vi "Pockels modulation-Gen AO seq for funct img.vi"(7 "Run as sub-VI":bool, 11 "Setup/Logging queue element":T8={"Imaging Protocol"=enum."Live Imaging", "Number of Trials"=0, "Frame Size"=512, "# Averaged frames"=0, "Dwell time (us)"=0.0, "Index of Z-plane"=0, "Timelapse?"=FALSE, "Logging process is active"=FALSE, "Speed logging enabled"=FALSE, "tdms file ref"=refnum, "path"=path "", "Trial Number"=0, "Expected # points acquired"=FALSE, "Manually stopped"=FALSE, "Last trial"=FALSE, "Ch0 data"=[], "Ch1 data"=[], "Ref Data"=[], "Ref Frame Time"=[], "Image Time"=[], "Continuous Time"=[], "Ref X Length"=0, "Ref Y Length"=0, "# Ref Averaged frames"=0, "Ref Dwell time (us)"=0.0, "Points acquired"={"Ch0 last trial"=0, "Ch1 last trial"=0, "All trials"=0}, "HW Timings File"=refnum} {"Ref Dwell time (us)" format="%#.6g"; "Frame Size" items=["100X100"=100, "128X128"=128, "200X200"=200, "256X256"=256, "512X512"=512, "1024x1024"=1024, "2048x2048"=2048]; "Dwell time (us)" format="%#.6g"}) -> (1 "Pockels modulation sequence":dbl[](array[numeric])=[0.0, 0.0, 0.0, 0.0, 0.0, 0.0, 0.0, 0.0, 0.0, 0.0, 0.0, 0.0, 0.0, 0.0, 0.0, 0.0, 0.0, 0.0, 0.0, 0.0, 0.0, 0.0, 0.48, 0.48, 0.48, 0.48, 0.48, 0.48, 0.0, 0.0, 0.0, 0.0, 0.0, 0.0, 0.0, 0.0, 0.0, 0.0, 0.0, 0.0, 0.0, 0.0, 0.0, 0.0, 0.0, 0.0, 0.5308080000000001, 0.5308080000000001, 0.5308080000000001, 0.5308080000000001, 0.5308080000000001, 0.5308080000000001, 0.0, 0.0, 0.0, 0.0, 0.0, 0.0, 0.0, 0.0, 0.0, 0.0, 0.0, 0.0, 0.0, 0.0, 0.0, 0.0, 0.0, 0.0, 0.0, 0.586992, 0.586992, 0.586992, 0.586992, 0.586992, 0.586992, 0.0, 0.0, 0.0, 0.0, 0.0, 0.0, 0.0, 0.0, 0.0, 0.0, 0.0, 0.0, 0.0, 0.0, 0.0, 0.0, 0.0, 0.0, 0.649124, 0.649124, 0.649124, 0.649124, 0.649124, 0.649124, 0.0, 0.0, 0.0, 0.0, 0.0, 0.0, 0.0, 0.0, 0.0, 0.0, 0.0, 0.0, 0.0, 0.0, 0.0, 0.0, 0.0, 0.0, 0.0, 0.717834, 0.717834, 0.717834, 0.717834, 0.717834, 0.717834, 0.0, 0.0, 0.0, 0.0, 0.0, 0.0, 0.0, 0.0, 0.0, 0.0, 0.0, 0.0, 0.0, 0.0, 0.0, 0.0, 0.0, 0.0, 0.793814, 0.793814, 0.793814, 0.793814, 0.793814, 0.793814, 0.0, 0.0, 0.0, 0.0, 0.0, 0.0, 0.0, 0.0, 0.0, 0.0, 0.0, 0.0, 0.0, 0.0, 0.0, 0.0, 0.0, 0.0, 0.0, 0.0, 0.0, 0.0, 0.0, 0.0, 0.0, 0.0, 0.0, 0.0, 0.0, 0.0, 0.0, 0.0, 0.0, 0.0, 0.0, 0.0, 0.0, 0.0, 0.0, 0.0, 0.0, 0.0, 0.0, 0.970756, 0.970756, 0.970756, 0.970756, 0.970756], 2 "Sampling period (us)":dbl=1e-06, 3 "Sequence length (ms)":dbl=198.0 format="%#_g ms", 4 "Sequence length (points)":i32=198 format="%.0f points")   [LabVIEW 2020]
uses:
  Typedefs/Logging queue element.ctl
  Typedefs/Imaging Protocols enum.ctl
  Typedefs/Frame Size.ctl
  Typedefs/Acquired points count.ctl
  Typedefs/Pockels-Funct acq simulation inputs cluster.ctl
  Typedefs/Controls/AOL_Globals.ctl
  Typedefs/AOL modes.ctl
  Typedefs/Plane Mode.ctl
  Typedefs/Functional Mode.ctl
  <vilib>/GPower/Comparison/Library/IsOdd/IsOddI32.vi
  <vilib>/GPower/Comparison/GPComparison.lvlib
panel:
  out "Last AOL_Globals used":T1={"Imaging Protocol"=enum."AOL Z-Stack", "Number of POI"=0, "Number of Miniscans"=0, "Number of Trials"=0, "Number of Cycles "=0, "# Averaged Frames"=0, "Laser power (%)"=0, "Pockels (V)"=0.0, "Acquisition Length (sec)"=0.0, "Fill time (us)"=0.0, "POI Dwell time (us)"=0.0, "Miniscan Dwell time per pixel (us)"=0.0, "PMT 1"=0.0, "PMT 2"=0.0, "Back Apperture (mA)"=200.0, "Frame Size"=0, "Center Frequency"=0.0, "Field of View (um)"=175.0, "Field of View (norm)"=0.0, "DwellTime (us)"=0.0, "Ref Dwell Time (us)"=0.0, "Wavelength (nm)"=0.0, "Zoom"=0.0, "AOL Z"=0.0, "AOL Mode"=enum."Raster", "GridXY"=0.0, "GridZ"=0.0, "TriggerPeriod (sec)"=0.0, "Number of Pixels in Miniscan"=0, "Experiment folder path"=path "", "X centre"=0.0, "Y centre"=0.0, "Angle (degrees)"=0.0, "Angle Xs (degrees)"=0.0, "Angle Ys (degrees)"=0.0, "Plane Mode"=0, "Threshold"=[], "Regenerate Chirps"=FALSE, "Rectangle ROI length (pixels)"=0, "Rectangle ROI height (pixels)"=0, "AOD fill"=4900, "StartupDelay"=0, "Samples Wait after Trigger"=5080, "Slip Cycle"=600000, "Add Cycle"=TRUE, "Functional Mode"=enum."Point", "Z Start"=0.0, "Z Stop"=0.0, "# Planes"=0, "Total Pixels"=0, "Variable Miniscan Pixels"=[], "Use Variable Length"=FALSE, "Use Variable Resolution"=FALSE, "Laser power (%) at Z Start"=0, "Laser power (%) at Z Stop"=0, "Ref Z Step"=0} {"Angle Ys (degrees)" format="%#.6g"; "Angle Xs (degrees)" format="%#.6g"; "Plane Mode" items=["XY Plane", "XZ Plane", "YZ Plane", "arbitraryplane"]; "Frame Size" items=["100X100"=100, "128X128"=128, "200X200"=200, "256X256"=256, "512X512"=512, "1024x1024"=1024, "2048x2048"=2048]; "Back Apperture (mA)" format="%#.6g"; "Pockels (V)" format="%#.6g"; "PMT 2" format="%#.6g"; "PMT 1" format="%#.6g"; "Angle (degrees)" format="%#.6g"; "POI Dwell time (us)" format="%#.6g"}
  in  "Temp Patch":bool=TRUE
  out "Loop":i32
  in  "Simulation inputs cluster":T7={"Dwell time (us) -Manual"=4.2, "Simulated number of POI"=80, "Bypass"=TRUE, "Movement Correction"=TRUE, "Ref_dwellTime"=0.1, "Ref X-pixels-per-line(Npxr)"=13, "Ref Y-lines-per-image(Npyr)"=12, "Ref Z-Plane index"=30, "Pockels \"Low\" time (us)"=20.0, "AO Sample Clock Rate (samples/sec)"=1000000.0, "Target time between mov.cor. ref triggers (ms)"=2.0, "Control system simulated waveform"=TRUE} {"AO Sample Clock Rate (samples/sec)" format="%#_6f"; "Dwell time (us) -Manual" min=0.05 max=10.0 step=0.1 format="%#.1fus"}
  out "Ref Scan Cycles":i32
  out "Adjusted time between ref \ntriggers sent to the FPGA (ms)":dbl
  in  "Pockels turn ON at least this number of us before fill time completion":dbl=4.0 min=0.05 max=10.0 step=1.0 format="%#.1fus"
  out "Number of POI":i32=8
  out "Cursor distance (us)":dbl=2.0 format="%#_g us"
  out "AO card sampling interval (us)":dbl=1.0 format="%#_13g us"
  out "Fill time (us)":dbl=24.4 format="%#_g us"
  in  "Pockels stay ON for at least this number of us after dwell time":dbl=2.0 min=0.5 max=10.0 step=1.0 format="%#.1fus"
  out "Graph":waveform(dbl)[](graph)=[{"t0"=timestamp(0 s since 1904-01-01), "dt"=0.05, "Y"=array[4561 elements]}, {"t0"=timestamp(0 s since 1904-01-01), "dt"=1.0, "Y"=[0.0, 0.0, 0.0, 0.0, 0.0, 0.0, 0.0, 0.0, 0.0, 0.0, 0.0, 0.0, 0.0, 0.0, 0.0, 0.0, 0.0, 0.0, 0.0, 0.0, 2.0, 2.0, 2.0, 2.0, 2.0, 2.0, 2.0, 2.0, 2.0, 2.0, 2.0, 2.0, 0.0, 0.0, 0.0, 0.0, 0.0, 0.0, 0.0, 0.0, 0.0, 0.0, 0.0, 0.0, 0.0, 0.0, 0.0, 0.0, 0.0, 2.0, 2.0, 2.0, 2.0, 2.0, 2.0, 2.0, 2.0, 2.0, 2.0, 2.0, 0.0, 0.0, 0.0, 0.0, 0.0, 0.0, 0.0, 0.0, 0.0, 0.0, 0.0, 0.0, 0.0, 0.0, 0.0, 0.0, 0.0, 2.0, 2.0, 2.0, 2.0, 2.0, 2.0, 2.0, 2.0, 2.0, 2.0, 2.0, 2.0, 0.0, 0.0, 0.0, 0.0, 0.0, 0.0, 0.0, 0.0, 0.0, 0.0, 0.0, 0.0, 0.0, 0.0, 0.0, 0.0, 0.0, 2.0, 2.0, 2.0, 2.0, 2.0, 2.0, 2.0, 2.0, 2.0, 2.0, 2.0, 0.0, 0.0, 0.0, 0.0, 0.0, 0.0, 0.0, 0.0, 0.0, 0.0, 0.0, 0.0, 0.0, 0.0, 0.0, 0.0, 0.0, 2.0, 2.0, 2.0, 2.0, 2.0, 2.0, 2.0, 2.0, 2.0, 2.0, 2.0, 2.0, 0.0, 0.0, 0.0, 0.0, 0.0, 0.0, 0.0, 0.0, 0.0, 0.0, 0.0, 0.0, 0.0, 0.0, 0.0, 0.0, 0.0, 2.0, 2.0, 2.0, 2.0, 2.0, 2.0, 2.0, 2.0, 2.0, 2.0, 2.0, 0.0, 0.0, 0.0, 0.0, 0.0, 0.0, 0.0, 0.0, 0.0, 0.0, 0.0, 0.0, 0.0, 0.0, 0.0, 0.0, 0.0, 2.0, 2.0, 2.0, 2.0, 2.0, 2.0, 2.0, 2.0, 2.0, 2.0, 2.0, 2.0, 0.0, 0.0, 0.0, 0.0, 0.0, 0.0, 0.0, 0.0, 0.0, 0.0, 0.0, 0.0, 0.0, 0.0, 0.0, 0.0, 0.0, 2.0, 2.0, 2.0, 2.0, 2.0, 2.0, 2.0]}]
  # "NOTE!\nThe always-simulated \"Control System\" signal may be wrong when Movement Correction is active as it won't include the reference frame time if\nthe number of POI result in very short original cycle time."
  # "<--- The pockels is an analogue signal which takes 3us to reach its value. Using 4us here ensures that the moment when data is acquired the pockels modulation signal has already reached its nominal value."
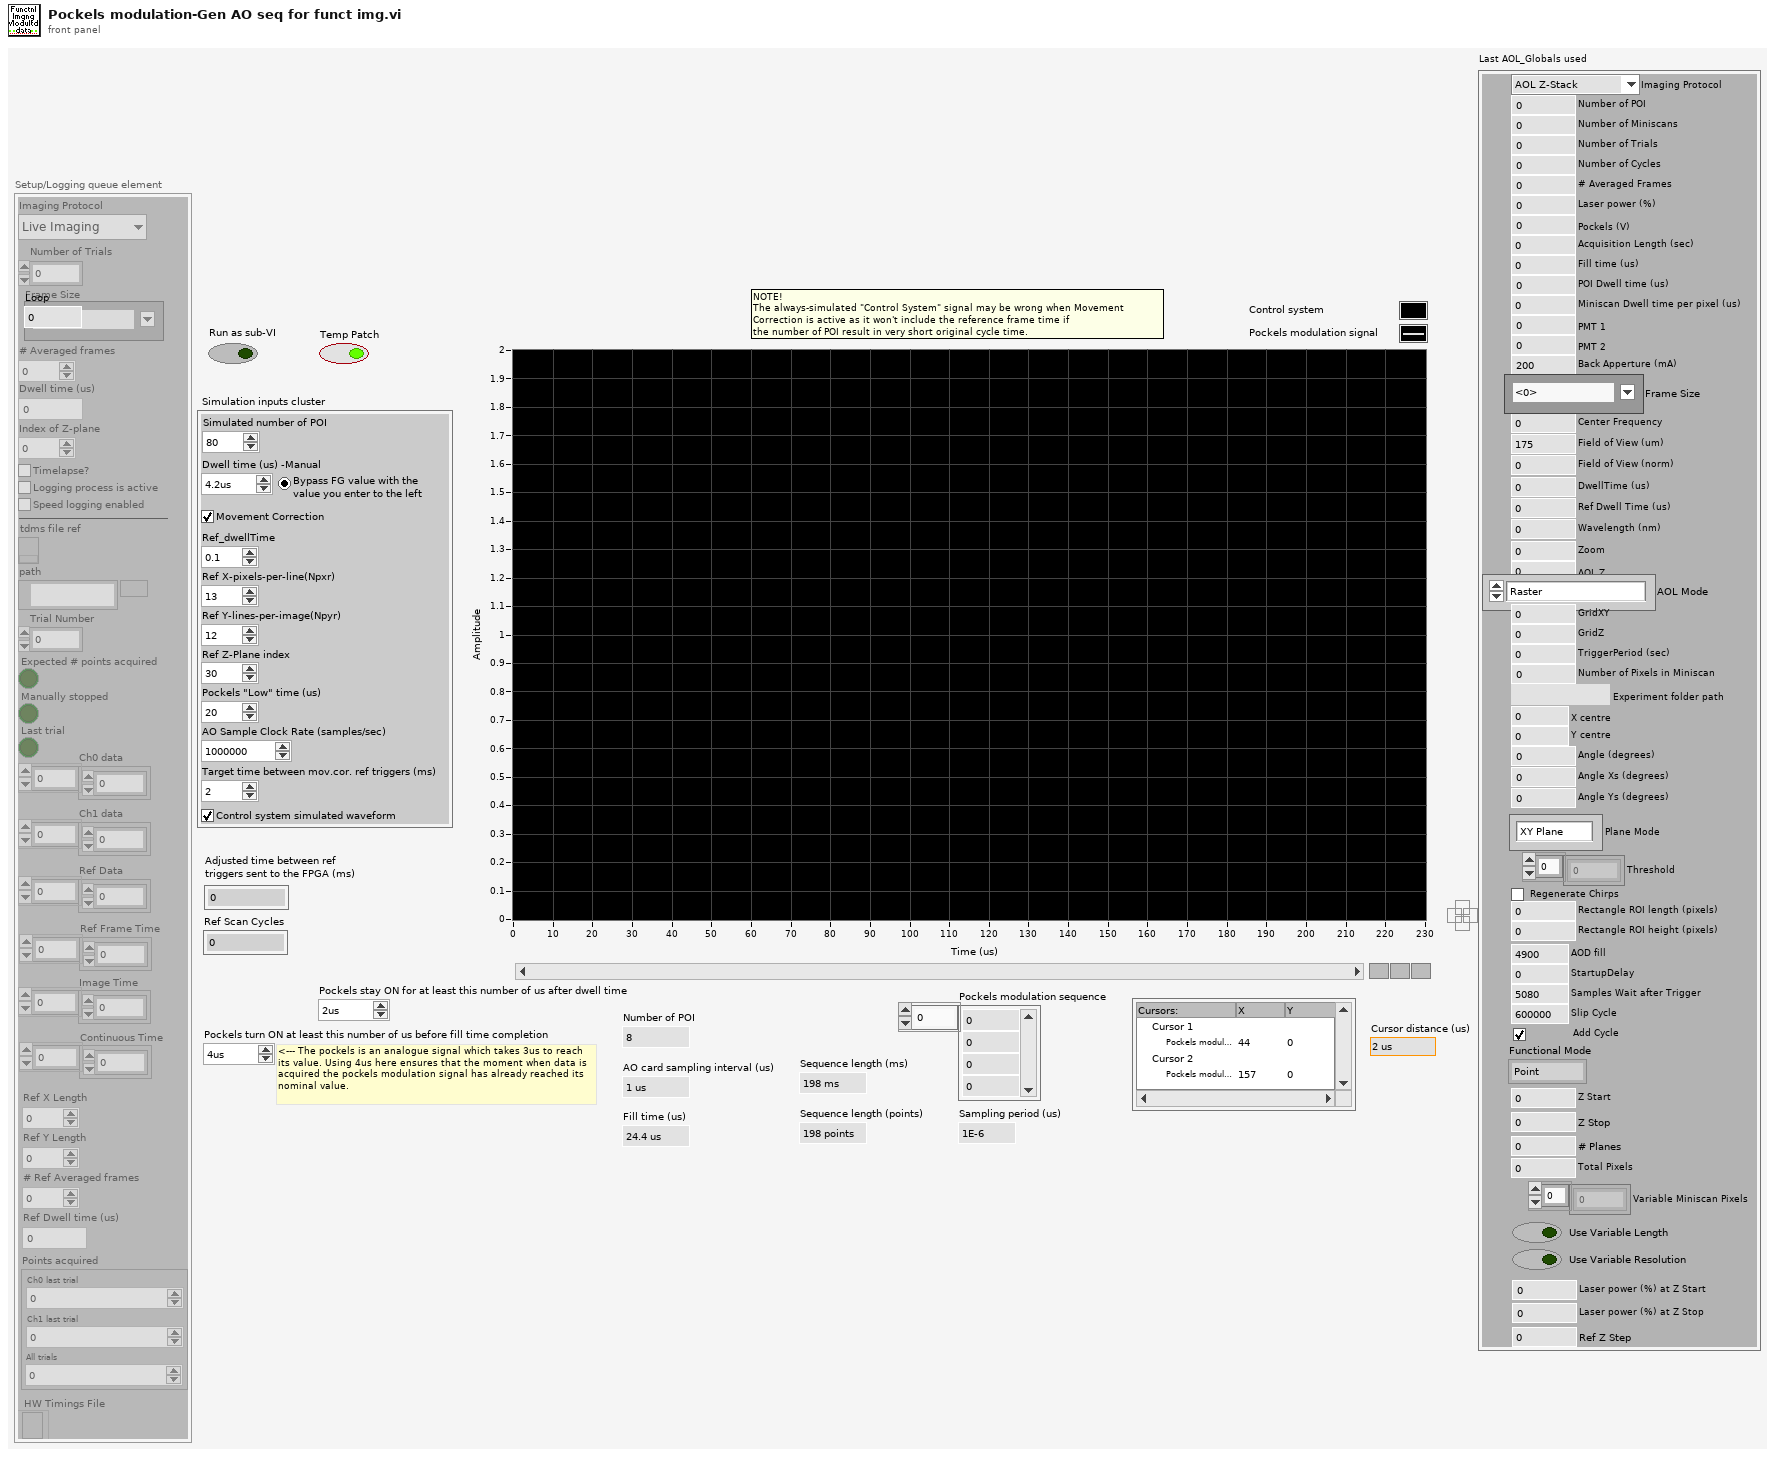
[diagram p1: front panel]
types:
  T1 = typedef "AOL_Globals.ctl" = cluster{"Imaging Protocol":T2, "Number of POI":u16, "Number of Miniscans":u16, "Number of Trials":u16, "Number of Cycles ":u64, "# Averaged Frames":u16, "Laser power (%)":u8, "Pockels (V)":dbl, "Acquisition Length (sec)":dbl, "Fill time (us)":dbl, "POI Dwell time (us)":dbl, "Miniscan Dwell time per pixel (us)":dbl, "PMT 1":dbl, "PMT 2":dbl, "Back Apperture (mA)":dbl, "Frame Size":T3, "Center Frequency":dbl, "Field of View (um)":dbl, "Field of View (norm)":dbl, "DwellTime (us)":dbl, "Ref Dwell Time (us)":dbl, "Wavelength (nm)":dbl, "Zoom":dbl, "AOL Z":dbl, "AOL Mode":T4, "GridXY":dbl, "GridZ":dbl, "TriggerPeriod (sec)":dbl, "Number of Pixels in Miniscan":u16, "Experiment folder path":path, "X centre":dbl, "Y centre":dbl, "Angle (degrees)":dbl, "Angle Xs (degrees)":dbl, "Angle Ys (degrees)":dbl, "Plane Mode":T5, "Threshold":u16[], "Regenerate Chirps":bool, "Rectangle ROI length (pixels)":u16, "Rectangle ROI height (pixels)":u16, "AOD fill":u16, "StartupDelay":i32, "Samples Wait after Trigger":u16, "Slip Cycle":u32, "Add Cycle":bool, "Functional Mode":T6, "Z Start":dbl, "Z Stop":dbl, "# Planes":i32, "Total Pixels":i32, "Variable Miniscan Pixels":u16[], "Use Variable Length":bool, "Use Variable Resolution":bool, "Laser power (%) at Z Start":u8, "Laser power (%) at Z Stop":u8, "Ref Z Step":i8}
  T2 = typedef "Imaging Protocols enum.ctl" = enum16{"AOL Z-Stack", "Motor Z Stack", "Parameter Sweep", "Functional Acquisition", "Single Plane Acquisition", "Volume Acquisition", "Live Imaging", "Live Plane Imaging", "Live Volume Imaging"}
  T3 = typedef "Frame Size.ctl" = u16
  T4 = typedef "AOL modes.ctl" = enum16{"Raster", "Structural", "Pointing", "Mini Scan", "Alignment"}
  T5 = typedef "Plane Mode.ctl" = u16
  T6 = typedef "Functional Mode.ctl" = enum16{"Point", "Line", "Patch", "Plane", "Volume"}
  T7 = typedef "Pockels-Funct acq simulation inputs cluster.ctl" = cluster{"Dwell time (us) -Manual":dbl, "Simulated number of POI":i32, "Bypass":bool, "Movement Correction":bool, "Ref_dwellTime":sgl, "Ref X-pixels-per-line(Npxr)":i16, "Ref Y-lines-per-image(Npyr)":i16, "Ref Z-Plane index":i32, "Pockels \"Low\" time (us)":dbl, "AO Sample Clock Rate (samples/sec)":dbl, "Target time between mov.cor. ref triggers (ms)":dbl, "Control system simulated waveform":bool}
  T8 = typedef "Logging queue element.ctl" = cluster{"Imaging Protocol":T2, "Number of Trials":u16, "Frame Size":T3, "# Averaged frames":u16, "Dwell time (us)":dbl, "Index of Z-plane":i32, "Timelapse?":bool, "Logging process is active":bool, "Speed logging enabled":bool, "tdms file ref":refnum<k34>, "path":path, "Trial Number":i32, "Expected # points acquired":bool, "Manually stopped":bool, "Last trial":bool, "Ch0 data":u32[], "Ch1 data":u32[], "Ref Data":u32[], "Ref Frame Time":u64[], "Image Time":u64[], "Continuous Time":u64[], "Ref X Length":u16, "Ref Y Length":u16, "# Ref Averaged frames":u16, "Ref Dwell time (us)":dbl, "Points acquired":T9, "HW Timings File":refnum<file>}
  T9 = typedef "Acquired points count.ctl" = cluster{"Ch0 last trial":u64, "Ch1 last trial":u64, "All trials":u64}
  T10 = typedef "ROI parameters data type.ctl" = cluster{"ROI index":dbl, "ROI ID":dbl, "ROI Time (ns)":dbl, "Pixels in ROI":dbl, "X start":dbl, "Y start":dbl, "Z start":dbl, "X stop":dbl, "Y stop":dbl, "Z stop":dbl, "Angle (deg)":dbl, "Composite ID":dbl, "Number of lines":dbl, "Frame Size":dbl, "Zoom":dbl, "Laser Power (%)":dbl, "ROI group ID":dbl, "Resolution":dbl, "Dwell Time per pixel":dbl, "Pixels per miniscan":dbl, "Original FOV (um)":dbl, "Apparent Frame Size":dbl, "Z Plane Idx":i32[], "Z Plane codes":i32[]}
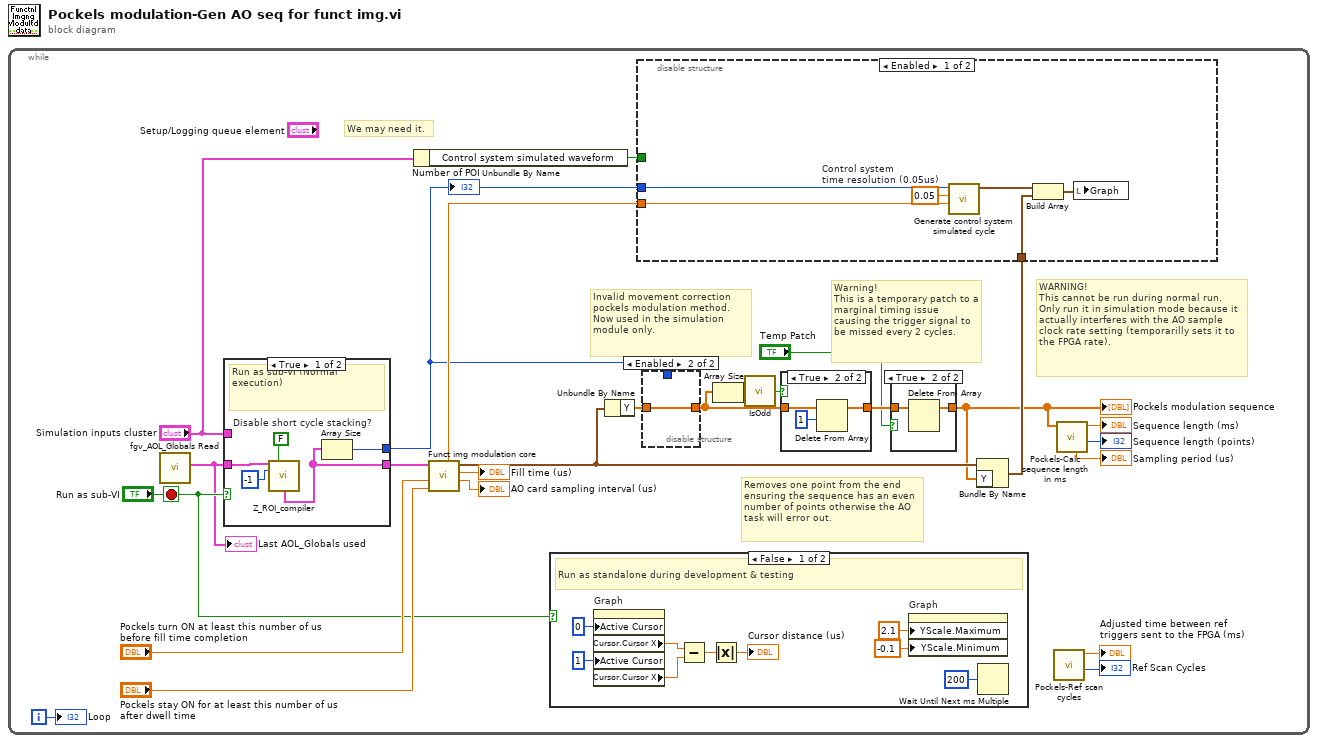
[diagram p0: block diagram]
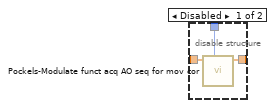
[diagram p3: hidden frame]
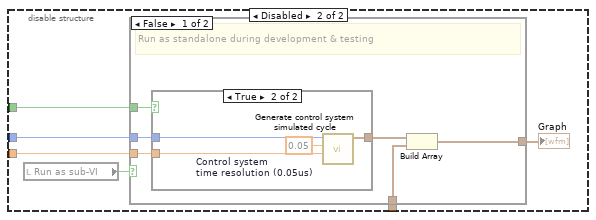
[diagram p4: hidden frame]
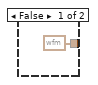
[diagram p5: hidden frame]
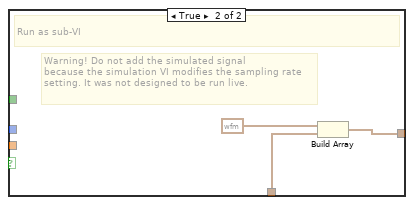
[diagram p6: hidden frame]
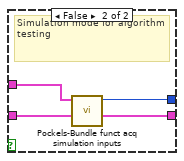
[diagram p7: hidden frame]
diagram:
  n1 = while {
    i -> [w6]
    stop <- "Run as sub-VI" stop-if-true
    # "Warning!\nThis is a temporary patch to a marginal timing issue \ncausing the trigger signal to be missed every 2 cycles."
    # "WARNING!\nThis cannot be run during normal run. Only run it in simulation mode because it actually interferes with the AO sample clock rate setting (temporarilly sets it to the FPGA rate)."
    # "Invalid movement correction pockels modulation method.\nNow used in the simulation module only."
    # "We may need it."
    # "Removes one point from the end ensuring the sequence has an even number of points otherwise the AO task will error out."
    n2 = call "fgv_AOL_Globals Read.vi"() -> ("AOL_Globals"=w1:T1)  [unwired: 9 in, 2 out]
    "Last AOL_Globals used" <- w1
    n3 = case shown="True" "Run as sub-VI" {
      tunnel: [w61 w67] -> w19
      tunnel: [w64 w68] -> w3
      tunnel: w1 -> [w63 w66]
      tunnel: "Simulation inputs cluster" -> [_ w65]
      frame True {
        w60 = FALSE  # Disable short cycle stacking?
        # "Run as sub-VI (Normal execution)"
        n4 = call "Z_ROI_compiler.vi"("AOL_Globals"=w63, "dISABLE"=w60, "Acquired z-plane index / volume index"=-1) -> ("ROI Attributes (broken down to miniscans)"=w61:T10[])  [unwired: 5 in, 7 out]
        n5 = Array Size(array=w61) -> (size(s)=w64:i32)
      }
      frame False {
        # "Simulation mode for algorithm testing"
        n6 = call "Pockels-Bundle funct acq simulation inputs.vi"("AOL_Globals"=w66, "Simulation inputs cluster"=w65) -> ("Array"=w67:T10[], "Simulated number of POI"=w68:i32)  [unwired: 8 in]
      }
    }
    "Number of POI" <- w3
    n7 = Unbundle By Name("Simulation inputs cluster") -> ("Control system simulated waveform"=w4:bool)
    n8 = call "Funct img modulation core.vi"("Pockels stay ON for at least this number of us after dwell time"="Pockels stay ON for at least this number of us after dwell time", "Pockels turn ON at least this number of us before fill time completion"="Pockels turn ON at least this number of us before fill time completion", "ROI setup"=w19) -> ("AO card sampling interval (us)"=→"AO card sampling interval (us)":dbl, "Fill time (us)"=→"Fill time (us)":dbl, "waveform out"=w15:waveform(dbl), "ROI Dwell Time (us)"=w16:dbl)  [unwired: 5 in]
    n9 = case shown="False" "Run as sub-VI" {
      frame False {
        # "Run as standalone during development & testing"
        n10 = property on="Graph" class="WFGraph (strict)"("Active Cursor"=u32 0, "Active Cursor"=u32 1) -> ("Cursor.Cursor X"=w78:dbl, "Cursor.Cursor X"=w77:dbl)  [unwired: 2 in, 2 out]
        n11 = Subtract(x=w78, y=w77) -> (x-y=w76:dbl)
        n12 = Absolute Value(x=w76) -> (abs(x)=→"Cursor distance (us)":dbl)
        n13 = property on="Graph" class="WFGraph (strict)"("YScale.Maximum"=2.1 ("Y Scale.Range:Maximum"), "YScale.Minimum"=-0.1 ("Y Scale.Range:Minimum")) -> ()  [unwired: 2 in, 2 out]
        n14 = Wait Until Next ms Multiple(millisecond multiple=u32 200) -> ()  [unwired: 1 out]
      }
      frame True {
        # "Run as sub-VI"
      }
    }
    n15 = Unbundle By Name(w15) -> ("Y"=w22:dbl[])
    n16 = disable-structure shown="Enabled" {
      disable-tunnel: w22 -> [w32 w33]
      disable-tunnel: [w31 w33] -> w21
      disable-tunnel: w3 -> [w30 _]
      frame Disabled {
        n17 = call "Pockels-Modulate funct acq AO seq for mov cor.vi"("Number of POI"=w30, "Pockels modulation sequence in"=w32) -> ("Pockels modulation sequence out"=w31:dbl[])  [unwired: 8 in, 1 out]
      }
      frame Enabled {
      }
    }
    n18 = Array Size(array=w21) -> (size(s)=w26:i32)
    n19 = call-poly <vilib>:"IsOdd.vi"("x"=w26) -> ("Odd?"=w25:bool)  [unwired: 4 in]
    n20 = case shown="True" w25 {
      tunnel: w21 -> [w69 w72]
      tunnel: [w69 w71] -> w24
      frame False {
      }
      frame True {
        n21 = Delete From Array(array=w72, length=1) -> (array with subset deleted=w71:dbl[])  [unwired: 1 in, 1 out]
      }
    }
    n22 = case shown="True" "Temp Patch" {
      tunnel: w24 -> [w27 w29]
      tunnel: [w27 w28] -> w12
      frame False {
      }
      frame True {
        n23 = Delete From Array(array=w29) -> (array with subset deleted=w28:dbl[])  [unwired: 2 in, 1 out]
      }
    }
    "Pockels modulation sequence" <- w12
    n24 = Bundle By Name(cluster=w15, "Y"=w12) -> (w23:waveform(dbl))
    n25 = disable-structure shown="Enabled" {
      disable-tunnel: w16 -> [w39 w45]
      disable-tunnel: w3 -> [w38 w44]
      disable-tunnel: w23 -> [w37 w43]
      disable-tunnel: w4 -> [_ w41]
      frame Enabled {
        w34 = 0.05  # Control system  time resolution (0.05us)
        n26 = call "Generate control system simulated cycle.vi"("ROI Dwell time (us)"=w39, "Control system time resolution (0.05us)"=w34, "Number of POI"=w38) -> ("Simulated control timings sequence (with Ref frames)"=w36:waveform(dbl))  [unwired: 7 in, 1 out]
        n27 = Build Array(w36, w37) -> (w35:waveform(dbl)[])
        n28 = local write "Graph"(w35) -> ()
      }
      frame Disabled {
        n29 = local read "Run as sub-VI"() -> (w42:bool)
        n30 = case shown="False" w42 {
          tunnel: w45 -> [w48 _]
          tunnel: w44 -> [w50 _]
          tunnel: w43 -> [w51 w58]
          tunnel: w41 -> [w49 _]
          tunnel: [w46 w59] -> w40
          frame False {
            # "Run as standalone during development & testing"
            n31 = case shown="True" w49 {
              tunnel: w48 -> [_ w56]
              tunnel: w50 -> [_ w55]
              tunnel: [waveform(dbl) {"t0"=timestamp(0 s since 1904-01-01), "dt"=1.0, "Y"=[]} ("element") w54] -> w47
              frame False {
              }
              frame True {
                w53 = 0.05  # Control system  time resolution (0.05us)
                n32 = call "Generate control system simulated cycle.vi"("ROI Dwell time (us)"=w56, "Control system time resolution (0.05us)"=w53, "Number of POI"=w55) -> ("Simulated control timings sequence (with Ref frames)"=w54:waveform(dbl))  [unwired: 7 in, 1 out]
              }
            }
            n33 = Build Array(w47, w51) -> (w46:waveform(dbl)[])
          }
          frame True {
            # "Warning! Do not add the simulated signal \nbecause the simulation VI modifies the sampling rate setting. It was not designed to be run live."
            # "Run as sub-VI"
            n34 = Build Array(waveform(dbl) {"t0"=timestamp(0 s since 1904-01-01), "dt"=1.0, "Y"=[]} ("Control system indicative cycle waveform"), w58) -> (w59:waveform(dbl)[])
          }
        }
        "Graph" <- w40
      }
    }
    n35 = call "Pockels-Ref scan cycles.vi"() -> ("Ref Scan Cycles"=→"Ref Scan Cycles":i32, "Adjusted time between ref \ntriggers sent to the FPGA (ms)"=→"Adjusted time between ref \ntriggers sent to the FPGA (ms)":dbl)  [unwired: 10 in]
    n36 = call "Pockels-Calc sequence length in ms.vi"("Pockels modulation sequence in"=w12) -> ("Sequence length (points)"=→"Sequence length (points)":i32, "Sequence length (ms)"=→"Sequence length (ms)":dbl, "Sampling period (us)"=→"Sampling period (us)":dbl)  [unwired: 8 in]
    "Loop" <- w6
  }
